vi "Top Level.vi"() -> ()   [LabVIEW 2020]
doc: "This template is for the Queued Message Handler design pattern.\n\nThe Event Handling Loop generates messages based on user interface actions.\n\nThe Message Handling Loop processes messages generated by the Event Handling Loop, or by other messages. The messages are string values, so new messages can be added easily to the Message Cases case structure in the Message Handling Loop. Each message cluster can also provide an optional value for Message Data, which is a variant that can be converted to whatever message-specific data is required."
uses:
  controls/UI Data.ctl
  support/Message Queue/Enqueue Message (Single).vi
  Global 1.vi
  <vilib>/Utility/file.llb/Write Delimited Spreadsheet (string).vi
  <vilib>/Utility/error.llb/Error Cluster From Error Code.vi
  <vilib>/ErrorRing/Error Ring.xnode
  support/Message Queue/Message Queue.lvlib
  support/User Event - Stop/User Event - Stop.lvlib
panel:
  in  "File Path":path
  in  "Preferences":bool
  in  "Tab Control":enum32{"Main", "New Scenario", "Run Scenario"}(tab)
  in  "New Scenario":bool
  in  "Run Scenario":bool
  in  "Table Control":string[][](table)
  in  "Save Scenario":bool
  in  "Return":bool
  in  "Quit":bool
  in  "Edit Scenario":bool
  in  "Play Button":bool
  in  "Media Stop Button":bool
  out "number (0 to 1)":dbl
  out "Display <Replace Me>":string
  in  "Exit":bool
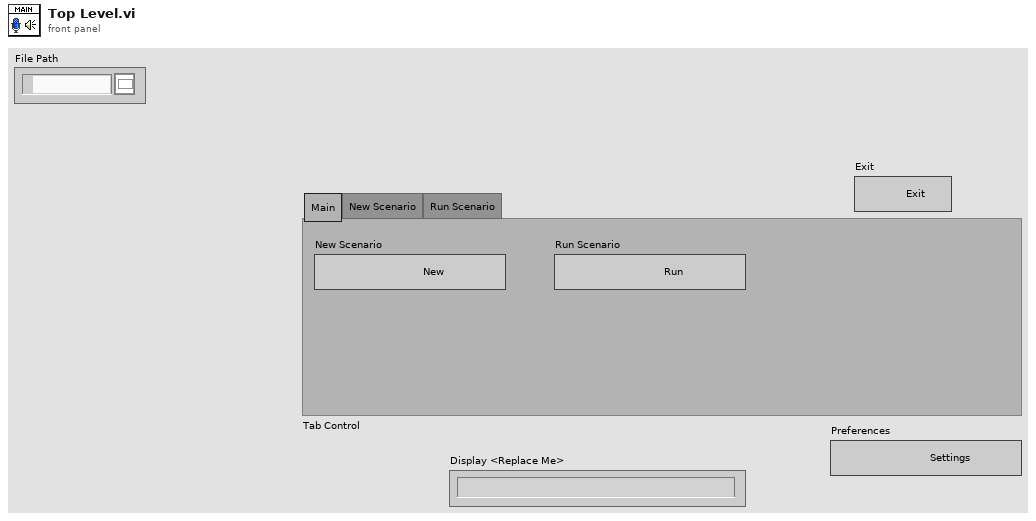
[diagram p1: front panel]
types:
  T1 = typedef "UI Data.ctl" = cluster{"Boolean <Replace Me>":bool, "String <Replace Me>":string, "Numeric <Replace Me>":dbl, "New Scenario Ref":refnum<vi>, "Run Scenario Else Ref":refnum<vi>, "Data Display Ref":refnum<vi>, "Exit Button Ref":refnum<vi>}
  T2 = typedef "Message Queue.lvlib/All Message Queues.ctl" = cluster{"UI":refnum<queue>}
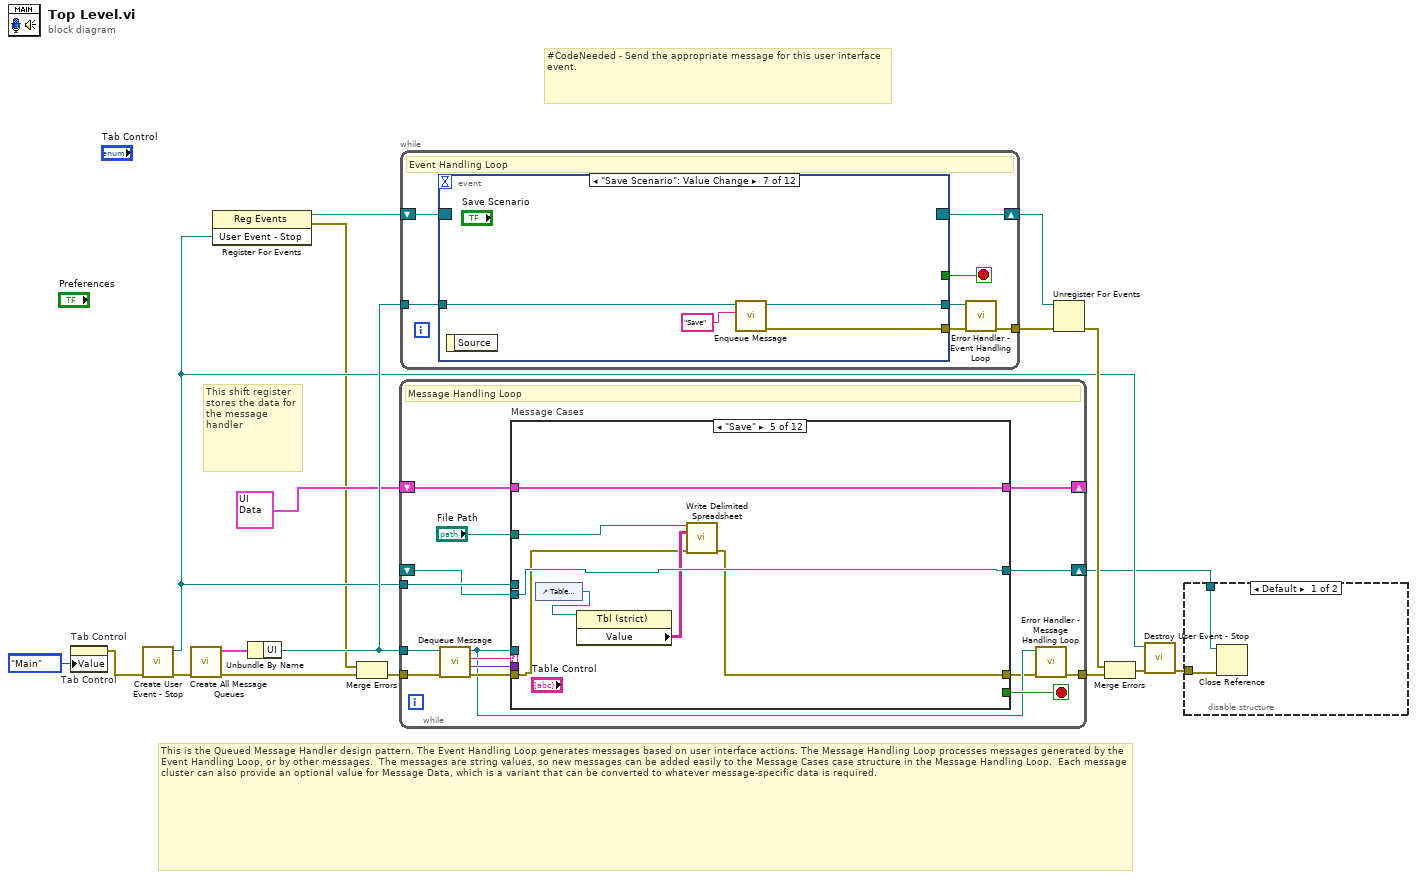
[diagram p0: block diagram]
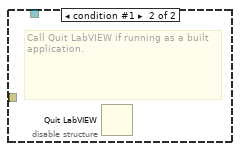
[diagram p2: hidden frame]
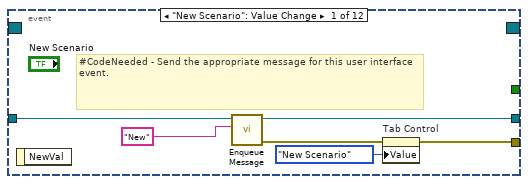
[diagram p3: hidden frame]
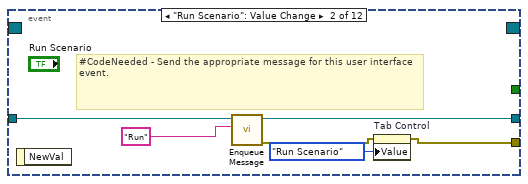
[diagram p4: hidden frame]
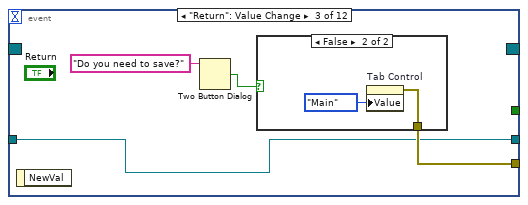
[diagram p5: hidden frame]
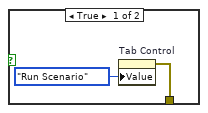
[diagram p6: hidden frame]
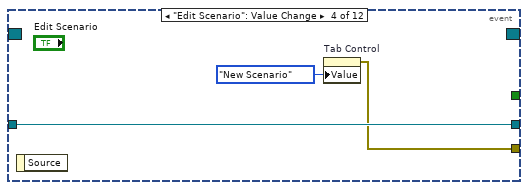
[diagram p7: hidden frame]
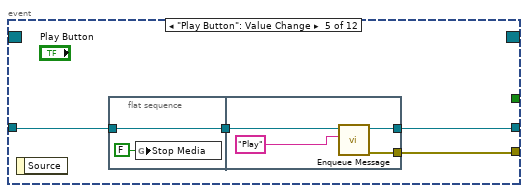
[diagram p8: hidden frame]
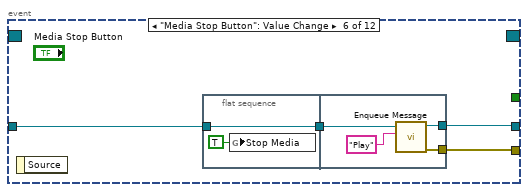
[diagram p9: hidden frame]
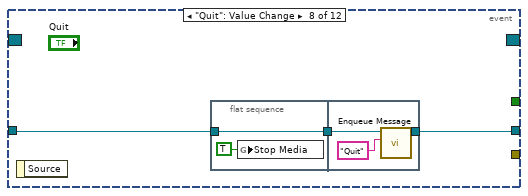
[diagram p10: hidden frame]
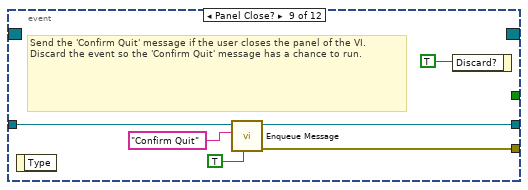
[diagram p11: hidden frame]
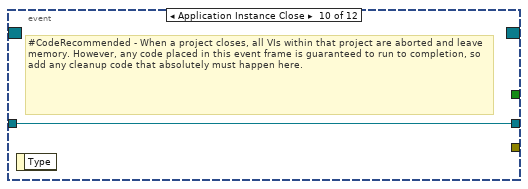
[diagram p12: hidden frame]
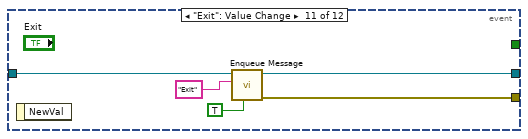
[diagram p13: hidden frame]
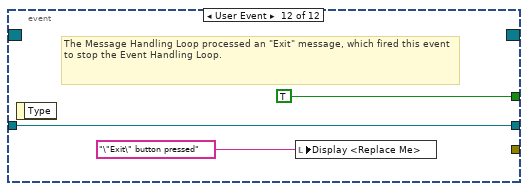
[diagram p14: hidden frame]
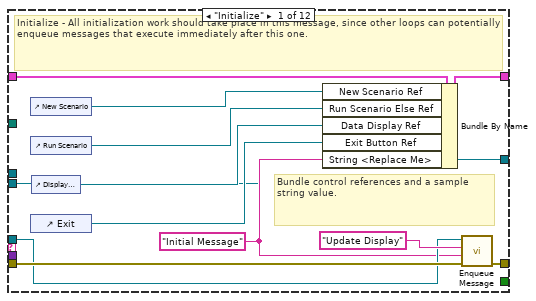
[diagram p15: hidden frame]
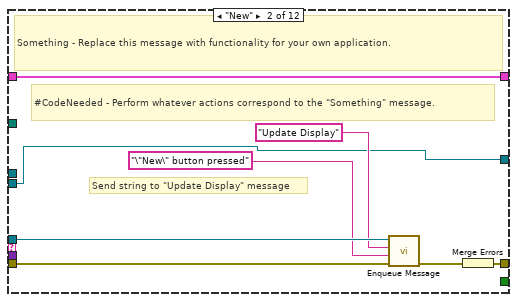
[diagram p16: hidden frame]
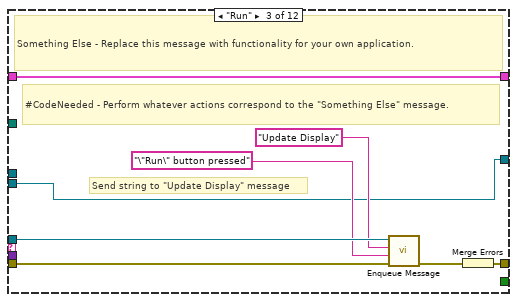
[diagram p17: hidden frame]
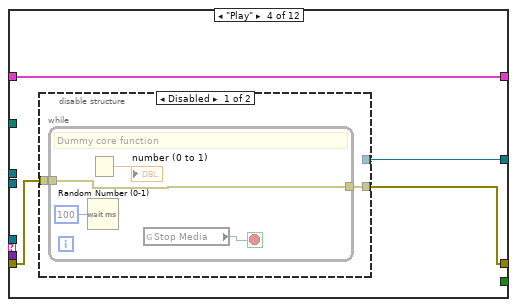
[diagram p18: hidden frame]
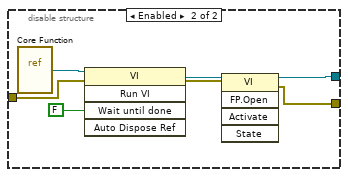
[diagram p19: hidden frame]
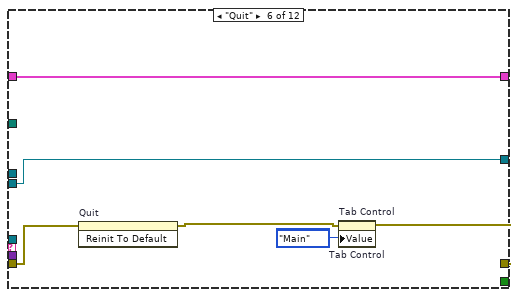
[diagram p20: hidden frame]
diagram:
  # "#CodeNeeded - Send the appropriate message for this user interface event."
  # "This is the Queued Message Handler design pattern. The Event Handling Loop generates messages based on user interface actions. The Message Handling Loop processes messages generated by the Event Handling Loop, or by other messages.  The messages are string values, so new messages can be added easily to the Message Cases case structure in the Message Handling Loop.  Each message cluster can also provide an optional value for Message Data, which is a variant that can be converted to whatever message-specific data is required."
  # "This shift register stores the data for the message handler"
  n1 = property on="Tab Control" class="TabCtl (strict)"("Value"=enum32{"Main", "New Scenario", "Run Scenario"}."Main" ("Tab Control")) -> ()  [unwired: 2 in, 2 out]
  n2 = property on="Tab Control" class="TabCtl (strict)"("Value"=enum32{"Main", "New Scenario", "Run Scenario"}."Main" ("Tab Control")) -> (error out=w3:errorcluster)  [unwired: 2 in, 1 out]
  n3 = call "Create User Event - Stop.vi"("error in (no error)"=w3) -> ("error out"=w15:errorcluster, "User Event - Stop"=w7:refnum<user-event>)  [unwired: 9 in]
  n4 = call "Create All Message Queues.vi"("error in (no error)"=w15) -> ("error out"=w19:errorcluster, "Message Queues out"=w18:T2)  [unwired: 9 in]
  n5 = register-events(w7) -> (reference out=w8:refnum<event-registration>, error out=w5:errorcluster)  [unwired: 2 in]
  n6 = Unbundle By Name(w18) -> ("UI"=w16:refnum<queue>)
  n7 = Merge Errors(w5, w19) -> (w6:errorcluster)
  n8 = while {
    tunnel: w16 -> [w26]
    shift-right: [w33] -> _
    shift-left: T1 {"Boolean <Replace Me>"=FALSE, "String <Replace Me>"="", "Numeric <Replace Me>"=0.0, "New Scenario Ref"=refnum, "Run Scenario Else Ref"=refnum, "Data Display Ref"=refnum, "Exit Button Ref"=refnum} ("Data Cluster") -> [w34]
    tunnel: w7 -> [w31]
    tunnel: w6 -> [w30]
    tunnel: [w24] -> w17
    shift-right: [w22] -> w1
    shift-left: _ -> [w21]
    stop <- w32 stop-if-true
    # "Message Handling Loop"
    n9 = call "Dequeue Message.vi"("error in (no error)"=w30, "Message Queue"=w26) -> ("error out"=w29:errorcluster, "Message Data"=w27:variant, "Message"=w28:string, "dup Message Queue"=w25:refnum<queue>)  [unwired: 6 in]
    n10 = case "Message Cases" shown="\"Save\"" w28 {
      selector: w28 -> [_ _ _ _ _ _ _ _ _ _ _ w135]
      tunnel: w25 -> [w37 w50 w58 _ _ _ _ _ w113 _ w133 _]
      tunnel: w29 -> [w45 w52 w60 w65 w81 w89 w99 w109 w117 w121 w127 _]
      tunnel: [w46 w53 w61 w64 w80 w90 w100 w103 w115 w119 w130 w136] -> w23
      tunnel: w34 -> [w44 w54 w62 w66 w86 w93 w101 w108 w116 w120 w132 w137]
      tunnel: [w43 w54 w62 w66 w86 w93 w101 w108 w116 w120 w132 w137] -> w33
      tunnel: [_ _ _ _ _ _ _ _ _ _ TRUE _] -> w32
      tunnel: w27 -> [_ _ _ _ _ _ w98 w107 _ _ w124 _]
      tunnel: w31 -> [_ _ _ _ _ _ _ _ _ _ w129 _]
      tunnel: [w35 w47 w55 w63 w84 w87 w94 w102 w110 w118 w123 w134] -> w22
      tunnel: w21 -> [w35 w47 w55 _ w84 w87 w94 w102 w110 w118 w123 w134]
      tunnel: "File Path" -> [_ _ _ _ w82 _ _ _ _ _ _ _]
      frame "Initialize" {
        w36 = "Initial Message" ("Initial Message")
        # "Bundle control references and a sample string value."
        # "Initialize - All initialization work should take place in this message, since other loops can potentially enqueue messages that execute immediately after this one."
        n11 = control-ref of="New Scenario"() -> (w42:refnum<vi>)
        n12 = control-ref of="Run Scenario"() -> (w41:refnum<vi>)
        n13 = control-ref of="Exit"() -> (w39:refnum<vi>)
        n14 = control-ref of="Display <Replace Me>"() -> (w40:refnum<vi>)
        n15 = Bundle By Name(cluster=w44, "New Scenario Ref"=w42, "Run Scenario Else Ref"=w41, "Data Display Ref"=w40, "Exit Button Ref"=w39, "String <Replace Me>"=w36) -> (w43:T1)
        n16 = call-poly "Enqueue Message.vi"("error in (no error)"=w45, "Message Data"=w36, "Message"="Update Display", "Message Queue"=w37) -> ("error out"=w46:errorcluster)  [unwired: 6 in, 1 out]
      }
      frame "New" {
        # "Send string to \"Update Display\" message"
        # "#CodeNeeded - Perform whatever actions correspond to the \"Something\" message."
        # "Something - Replace this message with functionality for your own application."
        n17 = call-poly "Enqueue Message.vi"("error in (no error)"=w52, "Message Data"="\"New\" button pressed" ("\"Do Something\" button pressed"), "Message"="Update Display", "Message Queue"=w50) -> ("error out"=w51:errorcluster)  [unwired: 6 in, 1 out]
        n18 = Merge Errors(w51) -> (w53:errorcluster)
      }
      frame "Run" {
        # "Send string to \"Update Display\" message"
        # "#CodeNeeded - Perform whatever actions correspond to the \"Something Else\" message."
        # "Something Else - Replace this message with functionality for your own application."
        n19 = call-poly "Enqueue Message.vi"("error in (no error)"=w60, "Message Data"="\"Run\" button pressed" ("\"Do Something Else\" button pressed"), "Message"="Update Display", "Message Queue"=w58) -> ("error out"=w59:errorcluster)  [unwired: 6 in, 1 out]
        n20 = Merge Errors(w59) -> (w61:errorcluster)
      }
      frame "Play" {
        n21 = disable-structure shown="Disabled" {
          disable-tunnel: w65 -> [w68 w78]
          disable-tunnel: [w67 w74] -> w64
          disable-tunnel: [_ w73] -> w63
          frame Disabled {
            n22 = while {
              tunnel: w68 -> [w70]
              tunnel: [w70] -> w67
              stop <- w69 stop-if-true
              # "Dummy core function"
              n23 = Wait (ms)(milliseconds to wait=u32 100) -> ()  [unwired: 1 out]
              n24 = Random Number (0-1)() -> (number: 0 to 1=→"number (0 to 1)":dbl)
              n25 = global read "Global 1.vi" "Stop Media"() -> (w69:bool)
            }
          }
          frame Enabled {
            n26 = vi-ref "Core Function.vi"() -> (w79:refnum<vi>)
            n27 = invoke class="VI" method="Run VI"(reference=w79, error in=w78, "Wait until done"=FALSE ("Activate?")) -> (reference out=w76:refnum<vi>, error out=w75:errorcluster)  [unwired: 2 in, 3 out]
            n28 = invoke class="VI" method="FP.Open"(reference=w76, error in=w75) -> (reference out=w73:refnum<vi>, error out=w74:errorcluster)  [unwired: 3 in, 3 out]
          }
        }
      }
      frame "Save" {
        n29 = control-ref of="Table Control"() -> (w85:refnum<vi>)
        n30 = property class="Tbl (strict)"(reference=w85) -> ("Value"=w83:string[][])  [unwired: 1 in, 2 out]
        n31 = call-poly <vilib>:"Write Delimited Spreadsheet.vi"("file path (dialog if empty)"=w82, "2D data"=w83, "error in (no error)"=w81) -> ("error out"=w80:errorcluster)  [unwired: 11 in, 1 out]
      }
      frame "Quit" {
        n32 = invoke on="Quit" class="Bool (strict)" method="Reinit To Default"(error in=w89) -> (error out=w88:errorcluster)  [unwired: 2 in, 2 out]
        n33 = property on="Tab Control" class="TabCtl (strict)"(error in=w88, "Value"=enum32{"Main", "New Scenario", "Run Scenario"}."Main" ("Tab Control")) -> (error out=w90:errorcluster)  [unwired: 1 in, 1 out]
        n34 = property on="Tab Control" class="TabCtl (strict)"("Value"=enum32{"Main", "New Scenario", "Run Scenario"}."Main" ("Tab Control")) -> ()  [unwired: 2 in, 2 out]
      }
      frame "Update Display" {
        # "#CodeRecommended - If you wish to decouple the Message Handling Loop from your user interface, consider creating User Events (like the \"Stop\" event in this VI) to message the Event Handling Loop whenever the user interface needs updating."
        # "Update Display - Convert the message data to a string to display in the Data Display indicator."
        n35 = Variant To Data(error in=w99, type="", Variant=w98) -> (data=→"Display <Replace Me>":string, error out=w96:errorcluster)
        n36 = Merge Errors(w96) -> (w100:errorcluster)
      }
      frame "Error" {
        # "#CodeRecommended - If you ever change the name of this \"Error\" message, you'll need to update the name in the Check Loop Error.vi as well."
        # "#CodeRecommended - Consider creating a system for logging errors in some way. These errors are for notification purposes only. Handling of specific errors should be performed in the message frames that generated the error."
        # "Error - Display an error dialog. This message is sent by the \"Error Handler\" VIs at the end of other loops in this application."
        n37 = Variant To Data(error in=w109, type=errorcluster {"status"=FALSE, "code"=0, "source"=""} ("error constant"), Variant=w107) -> (data=w105:errorcluster, error out=w104:errorcluster)
        n38 = call <vilib>:"Simple Error Handler.vi"("error in (no error)"=w105) -> ()  [unwired: 4 in, 5 out]
        n39 = Merge Errors(w104) -> (w103:errorcluster)
      }
      frame "Confirm Quit" {
        # "#CodeNeeded - If you want to provide an \"Are you sure\" dialog (or some other notification) before the application exits, place that code here. This message is typically sent from a Panel Close? event."
        # "Confirm Quit - Message that can confirm whether or not the user wants to exit the application."
        n40 = call-poly "Enqueue Message.vi"("Priority Message? (F)"=TRUE, "error in (no error)"=w117, "Message"="Exit", "Message Queue"=w113) -> ("error out"=w114:errorcluster)  [unwired: 6 in, 1 out]
        n41 = Merge Errors(w114) -> (w115:errorcluster)
      }
      frame "---Copy This Frame---" {
        # "Duplicate this frame when creating new messages.  Change this comment in the duplicated frame to describe this message."
        n42 = Merge Errors(w121) -> (w119:errorcluster)
      }
      frame "Exit" {
        # "Stop the VI"
        # "Release the message queue reference"
        # "#CodeNeeded - Add any required cleanup code here. Note that if 'Exit' was called as a result of an error, an error dialog will be displayed. Add any custom error handling for an 'Exit' condition here as well."
        # "Exit - Exit the application."
        n43 = Variant To Data(type=errorcluster {"status"=FALSE, "code"=0, "source"=""} ("error constant"), Variant=w124) -> (data=w125:errorcluster)  [unwired: 1 in, 1 out]
        n44 = call <vilib>:"Simple Error Handler.vi"("error in (no error)"=w125) -> ()  [unwired: 4 in, 5 out]
        n45 = call "Fire User Event - Stop.vi"("User Event - Stop"=w129) -> ("error out"=w128:errorcluster)  [unwired: 10 in]
        n46 = Release Queue(queue=w133, error in (no error)=w127) -> (error out=w122:errorcluster)  [unwired: 1 in, 2 out]
        n47 = Merge Errors(w128, w122) -> (w130:errorcluster)
      }
      frame Default {
        # "'Default' case only runs if there is a message that isn't defined in any of the other cases.  Output a programming error."
        n48 = xnode "Error Ring"("parameter 0"=w135) -> ("error out"=w136:errorcluster)
      }
    }
    n49 = call "Error Handler - Message Handling Loop.vi"("error in (no error)"=w23, "Message Queue"=w25) -> ("dup error in"=w24:errorcluster)  [unwired: 8 in, 1 out]
  }
  n50 = while {
    tunnel: w16 -> [w151]
    shift-right: [w149] -> w12
    shift-left: w8 -> [w150]
    tunnel: [w145] -> w9
    stop <- w147 stop-if-true
    # "Event Handling Loop"
    n51 = event shown="[6] \"Save Scenario\": Value Change" {
      selector: w150 -> [_ _ _ _ _ _ _ _ _ _ _ _]
      dyn-events: [_ _ _ _ _ _ _ _ _ _ _ _] -> w149
      timeout: _ -> [_ _ _ _ _ _ _ _ _ _ _ _]
      tunnel: [_ _ _ _ _ _ _ _ _ _ _ TRUE ("Discard?")] -> w147
      tunnel: w151 -> [w157 w163 w166 w174 w176 w188 w197 w200 w211 w213 w218 w221]
      tunnel: [w154 w159 w167 w172 w177 w185 w195 _ w210 _ w217 _] -> w148
      tunnel: [w156 w162 w166 w174 w178 w186 w198 w201 w209 w213 w216 w221] -> w146
      event "New Scenario": Value Change {
        # "#CodeNeeded - Send the appropriate message for this user interface event."
        n52 = event-data() -> ()  [unwired: 1 in, 1 out]
        n53 = call-poly "Enqueue Message.vi"("Message"="New", "Message Queue"=w157) -> ("error out"=w153:errorcluster, "dup Message Queue"=w156:refnum<queue>)  [unwired: 8 in]
        n54 = property on="Tab Control" class="TabCtl (strict)"(error in=w153, "Value"=enum32{"Main", "New Scenario", "Run Scenario"}."New Scenario" ("Tab Control")) -> (error out=w154:errorcluster)  [unwired: 1 in, 1 out]
      }
      event "Run Scenario": Value Change {
        # "#CodeNeeded - Send the appropriate message for this user interface event."
        n55 = event-data() -> ()  [unwired: 1 in, 1 out]
        n56 = call-poly "Enqueue Message.vi"("Message"="Run", "Message Queue"=w163) -> ("error out"=w160:errorcluster, "dup Message Queue"=w162:refnum<queue>)  [unwired: 8 in]
        n57 = property on="Tab Control" class="TabCtl (strict)"(error in=w160, "Value"=enum32{"Main", "New Scenario", "Run Scenario"}."Run Scenario" ("Tab Control")) -> (error out=w159:errorcluster)  [unwired: 1 in, 1 out]
      }
      event "Return": Value Change {
        n58 = event-data() -> ()  [unwired: 1 in, 1 out]
        n59 = Two Button Dialog(message="Do you need to save?") -> (T button?=w165:bool)  [unwired: 2 in]
        n60 = case shown="False" w165 {
          tunnel: [w169 w171] -> w167
          frame True {
            n61 = property on="Tab Control" class="TabCtl (strict)"("Value"=enum32{"Main", "New Scenario", "Run Scenario"}."Run Scenario" ("Tab Control")) -> (error out=w169:errorcluster)  [unwired: 2 in, 1 out]
          }
          frame False {
            n62 = property on="Tab Control" class="TabCtl (strict)"("Value"=enum32{"Main", "New Scenario", "Run Scenario"}."Main" ("Tab Control")) -> (error out=w171:errorcluster)  [unwired: 2 in, 1 out]
          }
        }
      }
      event "Edit Scenario": Value Change {
        n63 = event-data() -> ()  [unwired: 1 in, 1 out]
        n64 = property on="Tab Control" class="TabCtl (strict)"("Value"=enum32{"Main", "New Scenario", "Run Scenario"}."New Scenario" ("Tab Control")) -> (error out=w172:errorcluster)  [unwired: 2 in, 1 out]
      }
      event "Play Button": Value Change {
        n65 = event-data() -> ()  [unwired: 1 in, 1 out]
        n66 = flat-sequence {
          tunnel: w176 -> [w180]
          tunnel: [w180] -> w175
          tunnel: [w183] -> w178
          tunnel: [w182] -> w177
          tunnel: w175 -> [w181]
          frame #0 {
            n67 = global write "Global 1.vi" "Stop Media"(FALSE ("Stop Media")) -> ()
          }
          frame #1 {
            n68 = call-poly "Enqueue Message.vi"("Message"="Play", "Message Queue"=w181) -> ("error out"=w182:errorcluster, "dup Message Queue"=w183:refnum<queue>)  [unwired: 8 in]
          }
        }
      }
      event "Media Stop Button": Value Change {
        n69 = event-data() -> ()  [unwired: 1 in, 1 out]
        n70 = flat-sequence {
          tunnel: w188 -> [w189]
          tunnel: [w189] -> w187
          tunnel: w187 -> [w193]
          tunnel: [w192] -> w186
          tunnel: [w191] -> w185
          frame #0 {
            n71 = global write "Global 1.vi" "Stop Media"(TRUE ("Stop Media")) -> ()
          }
          frame #1 {
            n72 = call-poly "Enqueue Message.vi"("Message"="Play", "Message Queue"=w193) -> ("error out"=w191:errorcluster, "dup Message Queue"=w192:refnum<queue>)  [unwired: 8 in]
          }
        }
      }
      event "Save Scenario": Value Change {
        n73 = event-data() -> ()  [unwired: 1 in, 1 out]
        n74 = call-poly "Enqueue Message.vi"("Message"="Save", "Message Queue"=w197) -> ("error out"=w195:errorcluster, "dup Message Queue"=w198:refnum<queue>)  [unwired: 8 in]
      }
      event "Quit": Value Change {
        n75 = event-data() -> ()  [unwired: 1 in, 1 out]
        n76 = flat-sequence {
          tunnel: w200 -> [w203]
          tunnel: [w203] -> w199
          tunnel: [w205] -> w201
          tunnel: w199 -> [w204]
          frame #0 {
            n77 = global write "Global 1.vi" "Stop Media"(TRUE ("Stop Media")) -> ()
          }
          frame #1 {
            n78 = call-poly "Enqueue Message.vi"("Message"="Quit", "Message Queue"=w204) -> ("dup Message Queue"=w205:refnum<queue>)  [unwired: 8 in, 1 out]
          }
        }
      }
      event Panel Close? {
        # "Send the 'Confirm Quit' message if the user closes the panel of the VI. Discard the event so the 'Confirm Quit' message has a chance to run."
        n79 = event-data() -> ()  [unwired: 1 in, 1 out]
        n80 = call-poly "Enqueue Message.vi"("Priority Message? (F)"=TRUE, "Message"="Confirm Quit", "Message Queue"=w211) -> ("error out"=w210:errorcluster, "dup Message Queue"=w209:refnum<queue>)  [unwired: 7 in]
        n81 = event-data("Discard?"=TRUE) -> ()  [unwired: 1 in, 1 out]
      }
      event Application Instance Close {
        # "#CodeRecommended - When a project closes, all VIs within that project are aborted and leave memory. However, any code placed in this event frame is guaranteed to run to completion, so add any cleanup code that absolutely must happen here."
        n82 = event-data() -> ()  [unwired: 1 in, 1 out]
      }
      event "Exit": Value Change {
        n83 = event-data() -> ()  [unwired: 1 in, 1 out]
        n84 = call-poly "Enqueue Message.vi"("Priority Message? (F)"=TRUE, "Message"="Exit", "Message Queue"=w218) -> ("error out"=w217:errorcluster, "dup Message Queue"=w216:refnum<queue>)  [unwired: 7 in]
      }
      event User Event {
        # "The Message Handling Loop processed an \"Exit\" message, which fired this event to stop the Event Handling Loop."
        n85 = event-data() -> ()  [unwired: 1 in, 1 out]
        n86 = local write "Display <Replace Me>"("\"Exit\" button pressed" ("VI Stopped")) -> ()
      }
    }
    n87 = call "Error Handler - Event Handling Loop.vi"("error in (no error)"=w148, "Message Queue"=w146) -> ("dup error in"=w145:errorcluster)  [unwired: 8 in, 1 out]
  }
  n88 = Unregister For Events(event registration refnum=w12, error in=w9) -> (error out=w13:errorcluster)
  n89 = Merge Errors(w13, w17) -> (w14:errorcluster)
  n90 = call "Destroy User Event - Stop.vi"("error in (no error)"=w14, "User Event - Stop"=w7) -> ("error out"=w10:errorcluster)  [unwired: 9 in]
  n91 = disable-structure shown="Default" {
    disable-tunnel: w10 -> [w223 _]
    disable-tunnel: w1 -> [w222 _]
    frame condition #0 (active) {
      n92 = Close Reference(reference=w222, error in (no error)=w223) -> ()  [unwired: 1 out]
    }
    frame condition #1 {
      # "Call Quit LabVIEW if running as a built application."
      n93 = Quit LabVIEW() -> ()  [unwired: 1 in]
    }
  }
